vi "Adresse Geraet Kennung.vi"(8 "error in (no error)":errorcluster caption="Fehler (Eingang, kein Fehler)", 11 "mini8 Steuerung PNS Eingang":refnum<class "mini8 Steuerung PNS.lvclass">) -> (0 "error out":errorcluster caption="Fehler (Ausgang)", 2 "Adressen":cluster{i32[][], i32}, 3 "mini8 Steuerung PNS Ausgang":refnum<class "mini8 Steuerung PNS.lvclass">)   [LabVIEW 2020, in "mini8 Steuerung PNS.lvclass"]
uses:
  mini8 Steuerung PNS.lvclass
  D:/Software/LabVIEW/LV2020/Compact_LP/LP und Compact Standardprogramm/ObjektKlassen/Steuerung PNS/Steuerung PNS.lvclass
  AdressIndex.ctl
  Steuerung PNS.lvclass
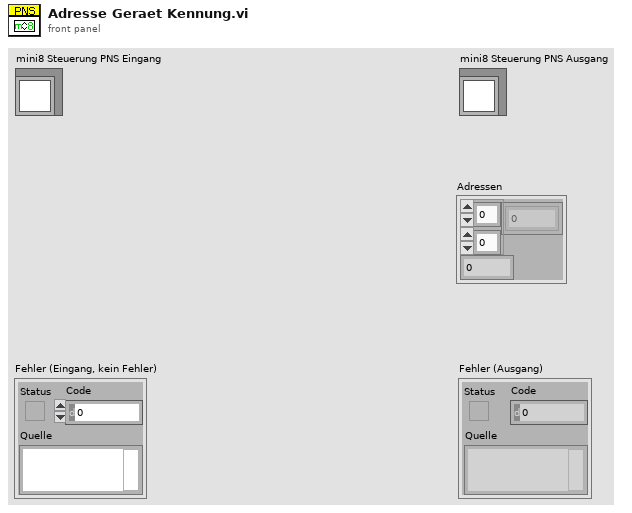
[diagram p1: front panel]
types:
  T1 = typedef "Steuerung PNS.lvclass/AdressIndex.ctl" = cluster{"Index":i32, "Index 2":i32, "Länge2":i32, "\nAnzahl":i32}
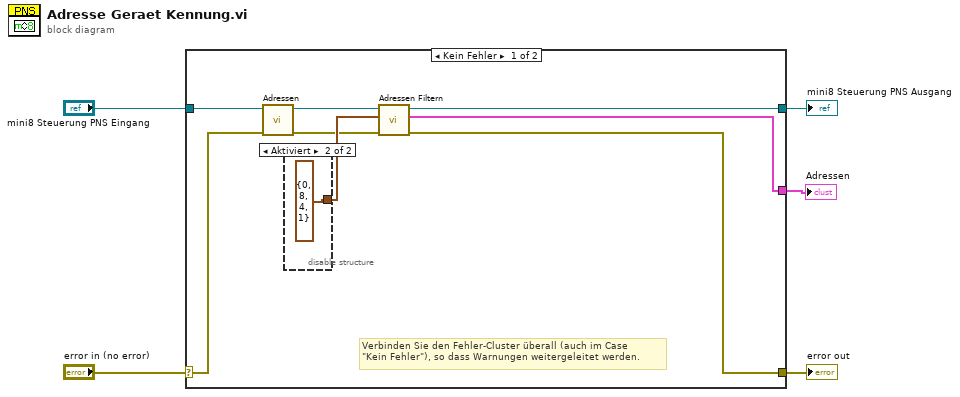
[diagram p0: block diagram]
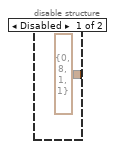
[diagram p2: hidden frame]
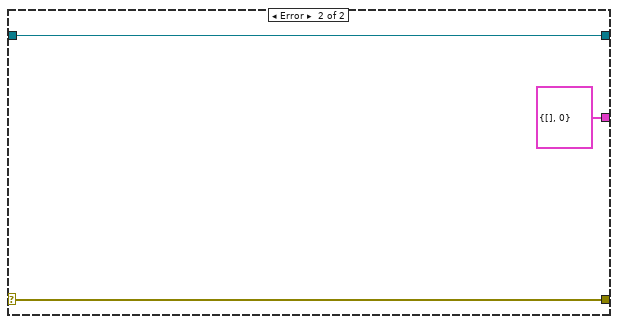
[diagram p3: hidden frame]
diagram:
  n1 = case shown="Kein Fehler" "error in (no error)" {
    selector: "error in (no error)" -> [w7 w18]
    tunnel: [w9 w18] -> w4
    tunnel: [w11 w17] -> w2
    tunnel: "mini8 Steuerung PNS Eingang" -> [w13 w17]
    tunnel: [w8 cluster{i32[][], i32} {[], 0} ("Adressen")] -> w1
    frame No Error {
      # "Verbinden Sie den Fehler-Cluster überall (auch im Case\n\"Kein Fehler\"), so dass Warnungen weitergeleitet werden."
      n2 = call-dynamic "Adressen.vi"("error in (no error)"=w7, "mini8 Steuerung PNS Eingang"=w13) -> ("error out"=w6:errorcluster, "mini8 Steuerung PNS Ausgang"=w12:refnum<class "mini8 Steuerung PNS.lvclass">)  [unwired: 7 in, 1 out]
      n3 = disable-structure shown="Aktiviert" {
        disable-tunnel: [T1 {"Index"=0, "Index 2"=8, "Länge2"=1, "\nAnzahl"=1} ("AdressIndex") T1 {"Index"=0, "Index 2"=8, "Länge2"=4, "\nAnzahl"=1} ("AdressIndex")] -> w10
        frame Disabled {
        }
        frame Enabled {
        }
      }
      n4 = call "Adressen Filtern.vi"("error in (no error)"=w6, "AdressIndex"=w10, "Steuerung PNS Eingang"=w12) -> ("error out"=w9:errorcluster, "Adressen"=w8:cluster{i32[][], i32}, "Steuerung PNS Ausgang"=w11:refnum<class "mini8 Steuerung PNS.lvclass">)  [unwired: 6 in]
    }
    frame Error {
    }
  }
  "error out" <- w4
  "mini8 Steuerung PNS Ausgang" <- w2
  "Adressen" <- w1
